vi "Tipo de señal.vi"() -> (3 "signal type":T1(ring))   [LabVIEW 2020, in "DataBase.lvlib"]
uses:
  DataBase.lvlib
  <vilib>/drjdpowell/SQLite Library/SQL Connection/Open (path).vi
  <vilib>/drjdpowell/SQLite Library/SQL Connection/Open (string).vi
  <vilib>/AdvancedString/Path To Command Line String.vi
  <vilib>/drjdpowell/SQLite Library/SQL Connection/Execute SQL (1D String).vi
  <vilib>/drjdpowell/SQLite Library/SQL Connection/Connection.lvclass
  <vilib>/drjdpowell/SQLite Library/SQLite.lvlib
panel:
  out "error out":errorcluster
  in  "error in (no error)":errorcluster
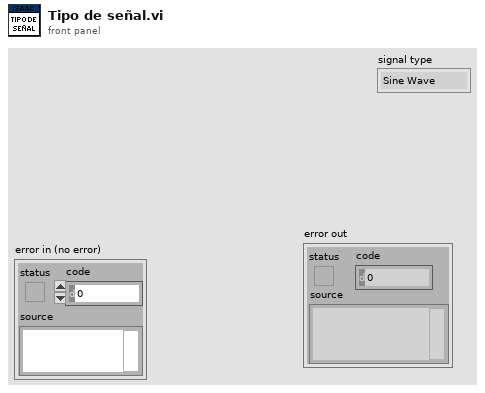
[diagram p1: front panel]
types:
  T1 = enum16{"Sine Wave", "Triangle Wave", "Square Wave", "Sawtooth Wave"}
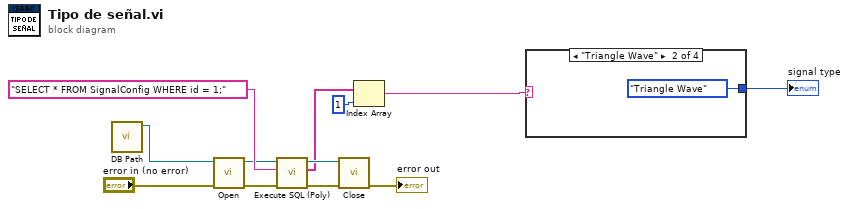
[diagram p0: block diagram]
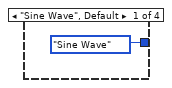
[diagram p2: hidden frame]
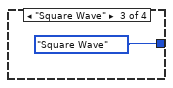
[diagram p3: hidden frame]
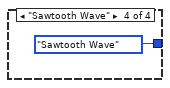
[diagram p4: hidden frame]
diagram:
  n1 = call "DB Path.vi"() -> ("appended path"=w1:path)  [unwired: 11 in]
  n2 = call-poly <vilib>:"Open.vi"("error in (no error)"="error in (no error)", "db file"=w1) -> ("error out"=w12:errorcluster, "SQLite Connection"=w5:refnum<class "Connection.lvclass">)  [unwired: 8 in]
  n3 = call-poly <vilib>:"Execute SQL (Poly).vi"("error in (no error)"=w12, "SQL"="SELECT * FROM SignalConfig WHERE id = 1;", "SQLite Connection in"=w5) -> ("error out"=w11:errorcluster, "Result Set"=w4:string[], "SQLite Connection"=w10:refnum<class "Connection.lvclass">)  [unwired: 5 in, 1 out]
  n4 = call-dynamic "Close.vi"("error in (no error)"=w11, "SQLite Connection in"=w10) -> ("error out"=→"error out":errorcluster)  [unwired: 9 in]
  n5 = Index Array(array=w4, index=1) -> (element=w3:string)
  n6 = case shown="\"Triangle Wave\"" w3 {
    tunnel: [T1."Sine Wave" ("signal type") T1."Triangle Wave" ("signal type") T1."Square Wave" ("signal type") T1."Sawtooth Wave" ("signal type")] -> w2
    frame "Sine Wave", Default {
    }
    frame "Triangle Wave" {
    }
    frame "Square Wave" {
    }
    frame "Sawtooth Wave" {
    }
  }
  "signal type" <- w2
